vi "SeCrTs-Hardware Config.vi"() -> ()   [LabVIEW 2022 SP3]
uses:
  Controls/SeCrTs-Config.ctl
panel:
  in  "Signal list":bool
  out "Config":T1={"AO config"=[], "AI config"=[], "DI config"=[], "DO config"=[], "TC config"=[{"Channel_Name"="", "Channel_Number"="", "Pre_Scale_min"=0.0, "Pre_Scale_max"=0.0, "units"=4, " type"=7}], "ACC config"=[], "SG config"=[], "Strain Gauge Settings"={"poisson ratio"=0.3, "nominal gage resistance"=120.0, "gage factor"=2.08}, "Bridge Settings"={"voltage excitation value"=3.3, "voltage excitation source"=10200, "initial bridge voltage"=0.0, "lead wire resistance"=1.7, "strain configuration"=10271}, "Sample Rate"={"AI Sample Rate"=[], "AO Sample Rate"=[], "DI Sample Rate"=[], "TC Sample Rate"=[], "DO Sample Rate"=[], "SG Sample Rate"=[], "ACC Sample Rate"=[]}} {"Bridge Settings"."strain configuration" items=["Full Bridge I"=10183, "Full Bridge II"=10184, "Full Bridge III"=10185, "Half Bridge I"=10188, "Half Bridge II"=10189, "Quarter Bridge I"=10271, "Quarter Bridge II"=10272]; "Bridge Settings"."voltage excitation source" items=["Internal"=10200, "External"=10167, "None"=10230]; "ACC config"."Terminal configuration" items=["default"=-1, "RSE"=10083, "NRSE"=10078, "Differential"=10106, "Pseudodifferential"=12529]; "ACC config"."Sensitivity units" items=["mVolts/g"=12509, "Volts/g"=12510]; "TC config"."type" items=["J"=10072, "K"=10073, "N"=10077, "R"=10082, "S"=10085, "T"=10086, "B"=10047, "E"=10055]; "TC config"."units" items=["Deg C", "Deg F", "Kelvins", "Deg R", "From Custom Scale"]}
  in  "Cancel":bool
  in  "Load Configuration":bool
  in  "New configuration":bool
  in  "Save Config":bool
  in  "Tab Control":T2(tab)
  in  "DO Sample Rate":dbl[](array[numeric]) format="%#_g Hz"
  in  "DO config":T3(array[cluster])=[{"Channel_Name"="", "Channel_Number"="", "Default_Value"=FALSE, "Units"=FALSE}]
  out "DO Device List":string[](array[string])
  in  "DI Sample Rate":dbl[](array[numeric]) format="%#_g Hz"
  in  "DI config":T3(array[cluster])
  out "DI Device List":string[](array[string])
  in  "AO Sample Rate":dbl[](array[numeric]) format="%#_g Hz"
  in  "AO config":T4(array[cluster])
  out "AO Device List":string[](array[string])
  in  "AI Sample Rate":dbl[](array[numeric]) format="%#_g Hz"
  in  "AI config":T5(array[cluster])
  out "AI Device List":string[](array[string])
  in  "TC Sample Rate":dbl[](array[numeric]) format="%#_g Hz"
  in  "TC config":T6(array[cluster]) {"thermocouple type" items=["J"=10072, "K"=10073, "N"=10077, "R"=10082, "S"=10085, "T"=10086, "B"=10047, "E"=10055]; "units" items=["Deg C"=10143, "Deg F"=10144, "Kelvins"=10325, "Deg R"=10145, "From Custom Scale"=10065]}
  out "TC Device List":string[](array[string])
  in  "ACC Sample Rate":dbl[](array[numeric]) format="%#_g Hz"
  in  "ACC config":T7(array[cluster]) {"Sensitivity units" items=["mVolts/g"=12509, "Volts/g"=12510]; "Terminal configuration" items=["default"=-1, "RSE"=10083, "NRSE"=10078, "Differential"=10106, "Pseudodifferential"=12529]}
  out "ACC Device List":string[](array[string])
  out "SG Device List":string[](array[string])
  in  "SG Sample Rate":dbl[](array[numeric]) format="%#_g Hz"
  in  "SG config":T8(array[cluster])
  in  "SG Settings":T9={"gage factor"=2.08, "nominal gage \nresistance"=120.0, "poisson ratio"=0.3}
  in  "Bridge Settings":T10={"voltage excitation value"=3.3, "voltage excitation source"=10200, "initial bridge voltage"=0.0, "lead wire resistance"=1.7, "strain configuration"=10271} {"strain configuration" items=["Full Bridge I"=10183, "Full Bridge II"=10184, "Full Bridge III"=10185, "Half Bridge I"=10188, "Half Bridge II"=10189, "Quarter Bridge I"=10271, "Quarter Bridge II"=10272]; "voltage excitation source" items=["Internal"=10200, "External"=10167, "None"=10230]}
  # "DO_Channel_Name"
  # "DO_Channel_Number"
  # "Default Value"
  # "Invert?"
  # "DI_Channel_Name"
  # "DI_Channel_Number"
  # "Default Value"
  # "Invert?"
  # "AO_Channel_Name"
  # "AO_Channel_Number"
  # "Default Value"
  # "Units"
  # "AI_Channel_Name"
  # "AI_Channel_Number"
  # "Pre_Scale_min"
  # "Pre_Scale_max"
  # "Scale_min"
  # "Scale_max"
  # "Units"
  # "TC_Channel_Name"
  # "TC_Channel_Number"
  # "Max_Value"
  # "Units"
  # "Type"
  # "Min_Value"
  # "ACC_Channel_Name"
  # "ACC_Channel_Number"
  # "Min_Value"
  # "Max_Value"
  # "Terminal Config"
  # "Sensitivity"
  # "Sensitivity Units"
  # "SG_Channel_Name"
  # "SG_Channel_Number"
  # "Min_Value"
  # "Max_Value"
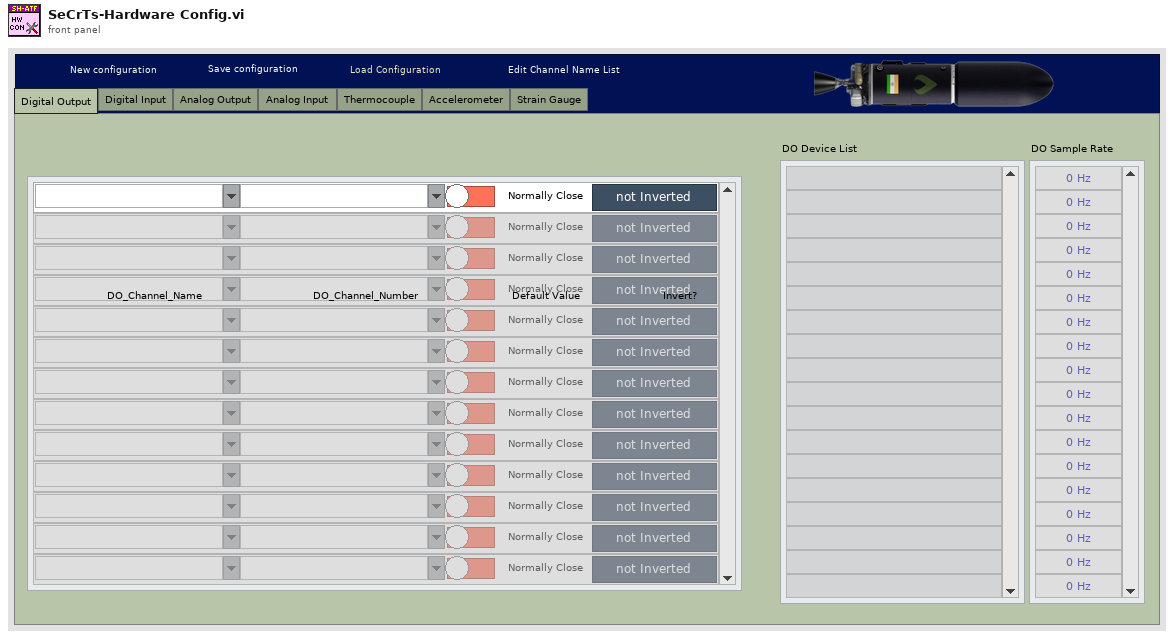
[diagram p1: front panel]
types:
  T1 = typedef "SeCrTs-Config.ctl" = cluster{"AO config":cluster{"Channel_Name":string, "Channel_Number":string, "Default_Value":dbl, "Units":string}[], "AI config":cluster{"Channel_Name":string, "Channel_Number":string, "Pre_Scale_min":dbl, "Pre_Scale_max":dbl, "Sensor_min":dbl, "Sensor_max":dbl, "Units":string}[], "DI config":cluster{"Channel_Name":string, "Channel_Number":string, "Default_Value":bool, "DI invert?":bool}[], "DO config":cluster{"Channel_Name":string, "Channel_Number":string, "Default_Value":bool, "DO invert?":bool}[], "TC config":cluster{"Channel_Name":string, "Channel_Number":string, "Pre_Scale_min":dbl, "Pre_Scale_max":dbl, "units":i32, " type":i32}[], "ACC config":cluster{"Channel_Name":string, "Channel_Number":string, "Pre_Scale_min":dbl, "Pre_Scale_max":dbl, "Terminal configuration":i32, "Sensitivity":dbl, "Sensitivity units":i32}[], "SG config":cluster{"Channel_Name":string, "Channel_Number":string, "Pre_Scale_min":dbl, "Pre_Scale_max":dbl}[], "Strain Gauge Settings":cluster{"poisson ratio":dbl, "nominal gage resistance":dbl, "gage factor":dbl}, "Bridge Settings":cluster{"voltage excitation value":dbl, "voltage excitation source":i32, "initial bridge voltage":dbl, "lead wire resistance":dbl, "strain configuration":i32}, "Sample Rate":cluster{"AI Sample Rate":dbl[], "AO Sample Rate":dbl[], "DI Sample Rate":dbl[], "TC Sample Rate":dbl[], "DO Sample Rate":dbl[], "SG Sample Rate":dbl[], "ACC Sample Rate":dbl[]}}
  T2 = enum32{"Digital Output", "Digital Input", "Analog Output", "Analog Input ", "Thermocouple", "Accelerometer", "Strain Gauge"}
  T3 = cluster{"Channel_Name":string, "Channel_Number":string, "Default_Value":bool, "Units":bool}[]
  T4 = cluster{"Channel_Name":string, "Channel_Number":string, "Default_Value":dbl, "Units":string}[]
  T5 = cluster{"Channel_Name":string, "Channel_Number":string, "Pre_Scale_min":dbl, "Pre_Scale_max":dbl, "Sensor_min":dbl, "Sensor_max":dbl, "Units":string}[]
  T6 = cluster{"Channel_Name":string, "Channel_Number":string, "Pre_Scale_min":dbl, "Pre_Scale_max":dbl, "units":i32, "thermocouple type":i32}[]
  T7 = cluster{"Channel_Name":string, "Channel_Number":string, "Pre_Scale_min":dbl, "Pre_Scale_max":dbl, "Terminal configuration":i32, "Sensitivity":dbl, "Sensitivity units":i32}[]
  T8 = cluster{"Channel_Name":string, "Channel_Number":string, "Pre_Scale_min":dbl, "Pre_Scale_max":dbl}[]
  T9 = cluster{"gage factor":dbl, "nominal gage \nresistance":dbl, "poisson ratio":dbl}
  T10 = cluster{"voltage excitation value":dbl, "voltage excitation source":i32, "initial bridge voltage":dbl, "lead wire resistance":dbl, "strain configuration":i32}
  T11 = cluster{"Device List":cluster{"AO Cards":tag[], "AI Cards":tag[], "DI Cards":tag[], "DO Cards":tag[]}, "Channel List":cluster{"AI Channel list":tag[], "AO Channel list":tag[], "DO Channel list ":tag[], "DI Channel list":tag[]}}
  T12 = cluster{"Channel List":cluster{"AI Channel list":tag[], "AO Channel list":tag[], "DO Channel list ":tag[], "DI Channel list":tag[]}, "Device List":cluster{"AO Cards":tag[], "AI Cards":tag[], "DI Cards":tag[], "DO Cards":tag[]}}
  T13 = cluster{"Data":T1, "path":path, "Name ref":refnum<vi>[], "Names":string[][], "Signal path":path, "SR":cluster{"AI Sample Rate":dbl[], "AO Sample Rate":dbl[], "DI Sample Rate":dbl[], "TC Sample Rate":dbl[], "DO Sample Rate":dbl[], "SG Sample Rate":dbl[], "ACC Sample Rate":dbl[]}, "Device List":cluster{"AO Cards":tag[], "AI Cards":tag[], "DI Cards":tag[], "DO Cards":tag[]}}
  T14 = typedef "SeCrTs-file folder ctl.ctl" = cluster{"Datalog path":path, "Configuration path":path, "Signal list path":path, "Sub vi's":path, "Authentication":path, "Sequence":path, "Event Log":path, "CS Error log":path, "RT Error Log":path}
  T15 = cluster{"AI":string[], "DI":string[], "DO":string[], "SG":string[], "AO":string[], "TC":string[], "ACC":string[]}
  T16 = cluster{"AI Channel list":tag[], "AO Channel list":tag[], "DO Channel list ":tag[], "DI Channel list":tag[]}
  T17 = cluster{"AO Cards":tag[], "AI Cards":tag[], "DI Cards":tag[], "DO Cards":tag[]}
  T18 = cluster{"AI Sample Rate":dbl[], "AO Sample Rate":dbl[], "DI Sample Rate":dbl[], "TC Sample Rate":dbl[], "DO Sample Rate":dbl[], "SG Sample Rate":dbl[], "ACC Sample Rate":dbl[]}
  T19 = enum16{"open", "replace", "create", "open or create", "replace or create", "replace or create with confirmation"}
  T20 = enum32{"Invalid", "Standard", "Closed", "Hidden", "Minimized", "Maximized"}
  T21 = cluster{"Channel_Name":string, "Channel_Number":string, "Default_Value":bool, "DI invert?":bool}[]
  T22 = cluster{"Channel_Name":string, "Channel_Number":string, "Default_Value":bool, "DO invert?":bool}[]
  T23 = cluster{"Channel_Name":string, "Channel_Number":string, "Pre_Scale_min":dbl, "Pre_Scale_max":dbl, "units":i32, " type":i32}[]
  T24 = cluster{"poisson ratio":dbl, "nominal gage resistance":dbl, "gage factor":dbl}
  T25 = cluster{"Channel_Name":string, "Channel_Number":string}
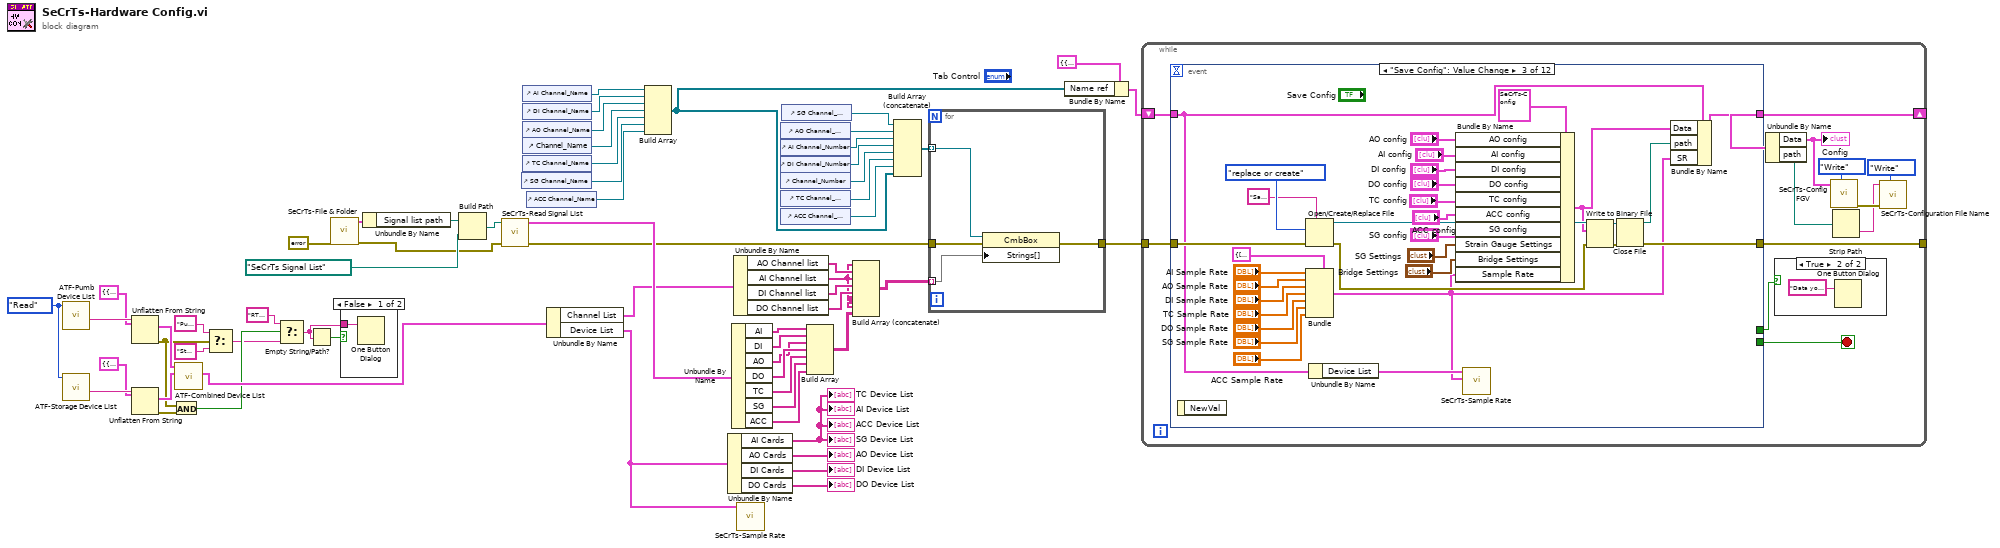
[diagram p0: block diagram]
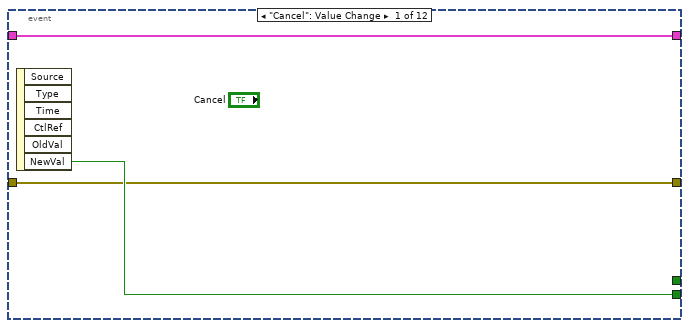
[diagram p4: hidden frame]
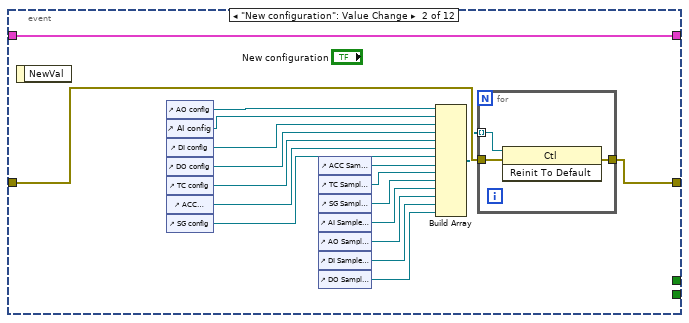
[diagram p5: hidden frame]
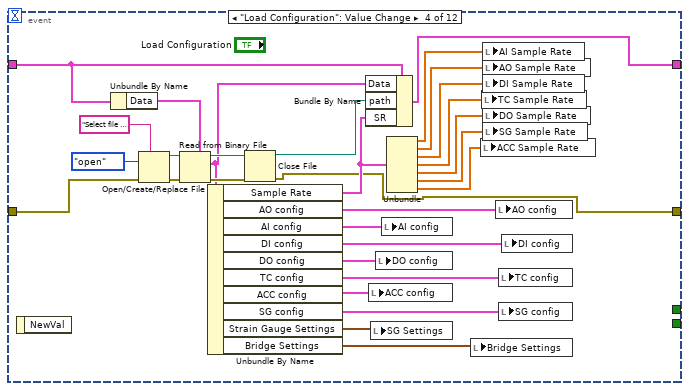
[diagram p6: hidden frame]
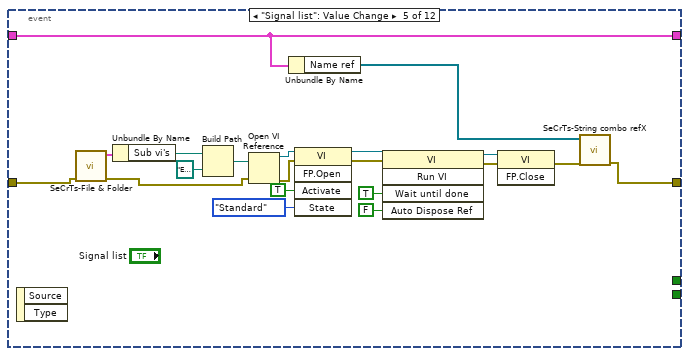
[diagram p7: hidden frame]
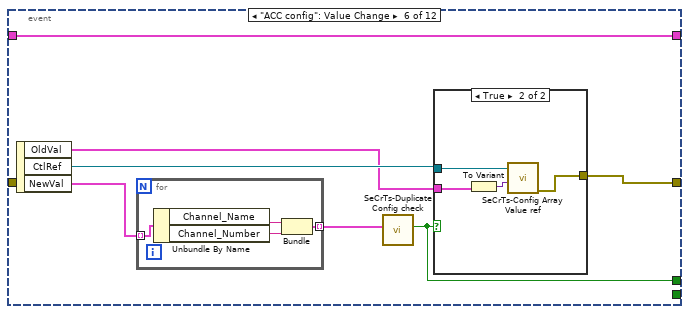
[diagram p8: hidden frame]
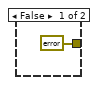
[diagram p9: hidden frame]
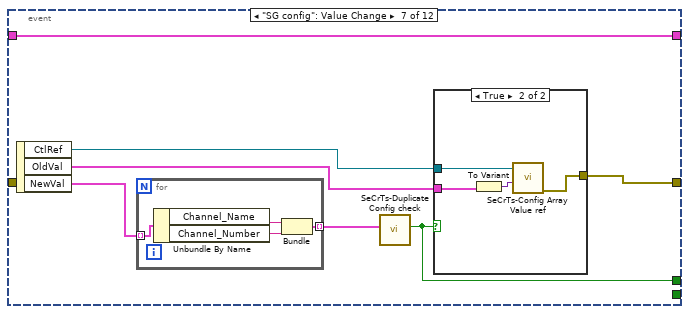
[diagram p10: hidden frame]
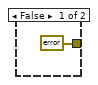
[diagram p11: hidden frame]
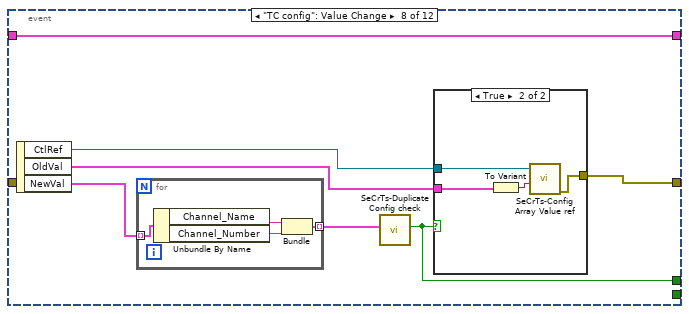
[diagram p12: hidden frame]
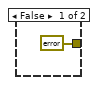
[diagram p13: hidden frame]
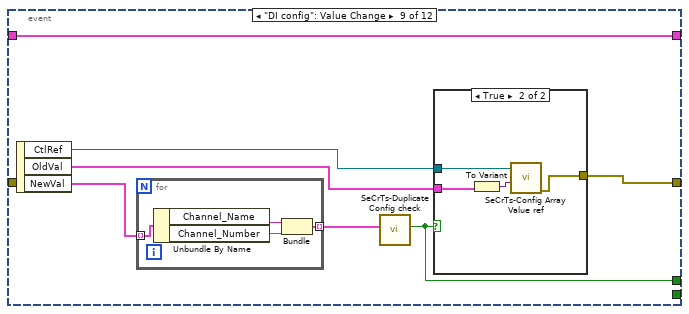
[diagram p14: hidden frame]
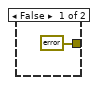
[diagram p15: hidden frame]
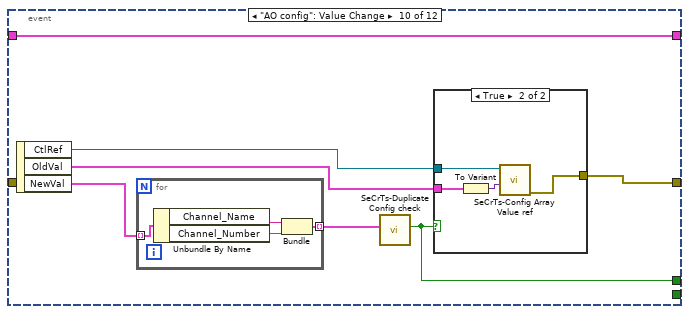
[diagram p16: hidden frame]
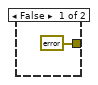
[diagram p17: hidden frame]
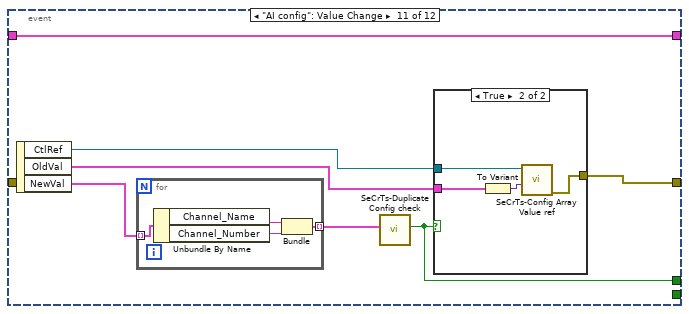
[diagram p18: hidden frame]
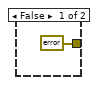
[diagram p19: hidden frame]
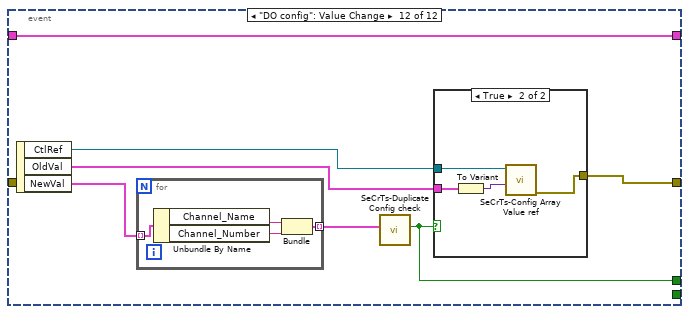
[diagram p20: hidden frame]
diagram:
  w16 = enum16{"Read", "Write", "Clear"}."Read" ("Enum")
  n1 = call "ATF-Pumb Device List.vi"("Enum"=w16) -> ("DL"=w15:string)  [unwired: 10 in]
  n2 = call "ATF-Storage Device List.vi"("Enum"=w16) -> ("DL"=w14:string)  [unwired: 10 in]
  n3 = Unflatten From String(type=T11 {"Device List"={"AO Cards"=[], "AI Cards"=[], "DI Cards"=[], "DO Cards"=[]}, "Channel List"={"AI Channel list"=[], "AO Channel list"=[], "DO Channel list "=[], "DI Channel list"=[]}}, binary string=w15) -> (value=w11:T11, error out=w6:errorcluster)  [unwired: 3 in, 1 out]
  n4 = Unflatten From String(type=T12 {"Channel List"={"AI Channel list"=[], "AO Channel list"=[], "DO Channel list "=[], "DI Channel list"=[]}, "Device List"={"AO Cards"=[], "AI Cards"=[], "DI Cards"=[], "DO Cards"=[]}}, binary string=w14) -> (value=w10:T12, error out=w9:errorcluster)  [unwired: 3 in, 1 out]
  n5 = And(x=w6, y=w9) -> (x .and. y?=w8:bool)
  n6 = call "ATF-Combined Device List.vi"("Storage"=w10, "Pump"=w11) -> ("Combined Device list"=w17:T12)  [unwired: 9 in]
  n7 = Select(t="Pump has heen not connected!" ("DL"), s=w6, f="Storage has heen not connected!" ("DL")) -> (s? t:f=w3:string)
  n8 = Select(t="RT has heen not connected!" ("DL"), s=w8, f=w3) -> (s? t:f=w2:string)
  n9 = Empty String/Path?(string/path=w2) -> (empty?=w1:bool)
  n10 = call "SeCrTs-File & Folder.vi"("error in (no error)"=errorcluster {"status"=FALSE, "code"=0, "source"=""} ("error in")) -> ("error out"=w42:errorcluster, "File Output"=w48:T14)  [unwired: 9 in]
  n11 = case shown="False" w1 {
    tunnel: w2 -> [w64 _]
    frame False {
      n12 = One Button Dialog(message=w64) -> ()  [unwired: 1 in, 1 out]
    }
    frame True {
    }
  }
  n13 = Unbundle By Name(w48) -> ("Signal list path"=w47:path)
  n14 = Build Path(base path=w47, name or relative path=path "SeCrTs Signal List") -> (appended path=w21:path)
  n15 = call "SeCrTs-Read Signal List.vi"("error in"=w42, "file path (use dialog)"=w21) -> ("error out"=w20:errorcluster, "Names"=w41:T15)  [unwired: 8 in]
  n16 = control-ref of="SG Channel_Name"() -> (w27:refnum<vi>)
  n17 = control-ref of="AI Channel_Name"() -> (w45:refnum<vi>)
  n18 = control-ref of="DI Channel_Name"() -> (w44:refnum<vi>)
  n19 = control-ref of="AO Channel_Name"() -> (w29:refnum<vi>)
  n20 = control-ref of="Channel_Name"() -> (w28:refnum<vi>)
  n21 = control-ref of="TC Channel_Name"() -> (w43:refnum<vi>)
  n22 = control-ref of="ACC Channel_Name"() -> (w26:refnum<vi>)
  n23 = Unbundle By Name(w17) -> ("Channel List"=w18:T16, "Device List"=w19:T17)
  n24 = Build Array(w45, w44, w29, w28, w43, w27, w26) -> (w30:refnum<vi>[])
  n25 = Unbundle By Name(w19) -> ("AI Cards"=→"AI Device List" →"TC Device List" →"ACC Device List" →"SG Device List":tag[], "AO Cards"=→"AO Device List":tag[], "DI Cards"=→"DI Device List":tag[], "DO Cards"=→"DO Device List":tag[])
  n26 = Unbundle By Name(w41) -> ("AI"=w40:string[], "DI"=w39:string[], "AO"=w34:string[], "DO"=w38:string[], "TC"=w37:string[], "SG"=w36:string[], "ACC"=w35:string[])
  n27 = Unbundle By Name(w18) -> ("AO Channel list"=w51:tag[], "AI Channel list"=w50:tag[], "DI Channel list"=w58:tag[], "DO Channel list"=w57:tag[])
  n28 = call "SeCrTs-Sample Rate.vi"("Device List"=w19) -> ()  [unwired: 11 in]
  n29 = control-ref of="AO Channel_Number"() -> (w63:refnum<vi>)
  n30 = control-ref of="AI Channel_Number"() -> (w62:refnum<vi>)
  n31 = control-ref of="DI Channel_Number"() -> (w61:refnum<vi>)
  n32 = control-ref of="Channel_Number"() -> (w60:refnum<vi>)
  n33 = control-ref of="TC Channel_Number"() -> (w54:refnum<vi>)
  n34 = control-ref of="ACC Channel_Number"() -> (w53:refnum<vi>)
  n35 = control-ref of="SG Channel_Number"() -> (w52:refnum<vi>)
  n36 = Build Array(w40, w39, w34, w38, w37, w36, w35) -> (w33:string[][])
  n37 = Build Array (concatenate)(w50, w51, w50, w58, w57, w50, w50, w33) -> (w56:string[][])
  n38 = Build Array (concatenate)(w52, w63, w62, w61, w60, w54, w53, w30) -> (w59:refnum<vi>[])
  n39 = for {
    tunnel: w59 -> [w68] mode=indexing
    tunnel: w56 -> [w65] mode=indexing
    tunnel: [w67] -> w55
    tunnel: w20 -> [w66]
    n40 = property class="CmbBox"(reference=w68, error in=w66, "Strings[]"=w65) -> (error out=w67:errorcluster)  [unwired: 1 out]
  }
  n41 = Bundle By Name(cluster=T13 {"Data"={"AO config"=[], "AI config"=[], "DI config"=[], "DO config"=[], "TC config"=[{"Channel_Name"="", "Channel_Number"="", "Pre_Scale_min"=0.0, "Pre_Scale_max"=0.0, "units"=4, " type"=7}], "ACC config"=[], "SG config"=[], "Strain Gauge Settings"={"poisson ratio"=0.3, "nominal gage resistance"=120.0, "gage factor"=2.08}, "Bridge Settings"={"voltage excitation value"=3.3, "voltage excitation source"=10200, "initial bridge voltage"=0.0, "lead wire resistance"=1.7, "strain configuration"=10271}, "Sample Rate"={"AI Sample Rate"=[], "AO Sample Rate"=[], "DI Sample Rate"=[], "TC Sample Rate"=[], "DO Sample Rate"=[], "SG Sample Rate"=[], "ACC Sample Rate"=[]}}, "path"=path "", "Name ref"=[], "Names"=[], "Signal path"=path "", "SR"={"AI Sample Rate"=[], "AO Sample Rate"=[], "DI Sample Rate"=[], "TC Sample Rate"=[], "DO Sample Rate"=[], "SG Sample Rate"=[], "ACC Sample Rate"=[]}, "Device List"={"AO Cards"=["PXI1Slot2"], "AI Cards"=["cDAQ1Mod1", "cDAQ1Mod2", "cDAQ1Mod3", "cDAQ1Mod4"], "DI Cards"=["cDAQ1Mod5", "PXI1Slot2", "PXI1Slot3"], "DO Cards"=["cDAQ1Mod5", "PXI1Slot2", "PXI1Slot3"]}}, "Name ref"=w30) -> (w32:T13)
  n42 = while {
    shift-right: [w76] -> _
    shift-left: w32 -> [w77]
    tunnel: w55 -> [w79]
    tunnel: [w78] -> _
    stop <- w80 stop-if-true
    n43 = event shown="[2] \"Save Config\": Value Change" {
      selector: _ -> [_ _ _ _ _ _ _ _ _ _ _ _]
      dyn-events: _ -> [_ _ _ _ _ _ _ _ _ _ _ _]
      timeout: _ -> [_ _ _ _ _ _ _ _ _ _ _ _]
      tunnel: [w83 _ _ _ _ _ _ _ _ _ _ _] -> w80
      tunnel: w79 -> [w82 w102 w137 w167 w187 _ _ _ _ _ _ _]
      tunnel: [w82 w101 w133 w144 w169 w189 w207 w223 w239 w255 w271 w287] -> w78
      tunnel: w77 -> [w84 w100 w109 w158 w172 w194 w210 w226 w242 w258 w274 w290]
      tunnel: [w84 w100 w125 w159 w172 w194 w210 w226 w242 w258 w274 w290] -> w76
      tunnel: [_ _ _ _ _ w188 w204 w220 w236 w252 w268 w284] -> w72
      event "Cancel": Value Change {
        n44 = event-data() -> ("NewVal"=w83:bool)  [unwired: 1 in, 5 out]
      }
      event "New configuration": Value Change {
        n45 = event-data() -> ()  [unwired: 1 in, 1 out]
        n46 = control-ref of="AO config"() -> (w95:refnum<vi>)
        n47 = control-ref of="AI config"() -> (w96:refnum<vi>)
        n48 = control-ref of="DI config"() -> (w97:refnum<vi>)
        n49 = control-ref of="DO config"() -> (w98:refnum<vi>)
        n50 = control-ref of="TC config"() -> (w94:refnum<vi>)
        n51 = control-ref of="ACC config"() -> (w93:refnum<vi>)
        n52 = control-ref of="SG config"() -> (w92:refnum<vi>)
        n53 = control-ref of="ACC Sample Rate"() -> (w91:refnum<vi>)
        n54 = control-ref of="TC Sample Rate"() -> (w90:refnum<vi>)
        n55 = control-ref of="SG Sample Rate"() -> (w89:refnum<vi>)
        n56 = control-ref of="AI Sample Rate"() -> (w88:refnum<vi>)
        n57 = control-ref of="AO Sample Rate"() -> (w87:refnum<vi>)
        n58 = control-ref of="DI Sample Rate"() -> (w86:refnum<vi>)
        n59 = control-ref of="DO Sample Rate"() -> (w85:refnum<vi>)
        n60 = Build Array(w95, w96, w97, w98, w94, w93, w92, w91, w90, w89, w88, w87, w86, w85) -> (w99:refnum<vi>[])
        n61 = for {
          tunnel: w99 -> [w105] mode=indexing
          tunnel: w102 -> [w104]
          tunnel: [w103] -> w101
          n62 = invoke class="Ctl" method="Reinit To Default"(reference=w105, error in=w104) -> (error out=w103:errorcluster)  [unwired: 1 in, 2 out]
        }
      }
      event "Save Config": Value Change {
        n63 = event-data() -> ()  [unwired: 1 in, 1 out]
        n64 = Open/Create/Replace File(error in=w137, prompt="Save Changes", operation (0:open)=T19."replace or create") -> (refnum out=w132:refnum<file>, error out=w136:errorcluster)  [unwired: 3 in, 1 out]
        n65 = Bundle(cluster=T18 {"AI Sample Rate"=[], "AO Sample Rate"=[], "DI Sample Rate"=[], "TC Sample Rate"=[], "DO Sample Rate"=[], "SG Sample Rate"=[], "ACC Sample Rate"=[]} ("Sample Rate"), "AI Sample Rate"="AI Sample Rate", "AO Sample Rate"="AO Sample Rate", "DI Sample Rate"="DI Sample Rate", "TC Sample Rate"="TC Sample Rate", "DO Sample Rate"="DO Sample Rate", "SG Sample Rate"="SG Sample Rate", "ACC Sample Rate"="ACC Sample Rate") -> (w107:T18)
        n66 = Unbundle By Name(w109) -> ("Device List"=w108:T17)
        n67 = Bundle By Name(cluster=T1 {"AO config"=[], "AI config"=[], "DI config"=[], "DO config"=[], "TC config"=[{"Channel_Name"="", "Channel_Number"="", "Pre_Scale_min"=0.0, "Pre_Scale_max"=0.0, "units"=4, " type"=7}], "ACC config"=[], "SG config"=[], "Strain Gauge Settings"={"poisson ratio"=0.3, "nominal gage resistance"=120.0, "gage factor"=2.08}, "Bridge Settings"={"voltage excitation value"=3.3, "voltage excitation source"=10200, "initial bridge voltage"=0.0, "lead wire resistance"=1.7, "strain configuration"=10271}, "Sample Rate"={"AI Sample Rate"=[], "AO Sample Rate"=[], "DI Sample Rate"=[], "TC Sample Rate"=[], "DO Sample Rate"=[], "SG Sample Rate"=[], "ACC Sample Rate"=[]}} ("Data"), "AO config"="AO config", "AI config"="AI config", "DI config"="DI config", "DO config"="DO config", "TC config"="TC config", "ACC config"="ACC config", "SG config"="SG config", "Strain Gauge Settings"="SG Settings", "Bridge Settings"="Bridge Settings", "Sample Rate"=w107) -> (w106:T1)
        n68 = call "SeCrTs-Sample Rate.vi"("Sample Rate"=w107, "Device List"=w108) -> ()  [unwired: 10 in]
        n69 = Write to Binary File(file (use dialog)=w132, data=w106, error in=w136) -> (refnum out=w135:refnum<file>, error out=w134:errorcluster)  [unwired: 3 in, 1 out]
        n70 = Close File(refnum=w135, error in=w134) -> (path=w120:path, error out=w133:errorcluster)
        n71 = Bundle By Name(cluster=w109, "Data"=w106, "path"=w120, "SR"=w107) -> (w125:T13)
      }
      event "Load Configuration": Value Change {
        n72 = event-data() -> ()  [unwired: 1 in, 1 out]
        n73 = Unbundle By Name(w158) -> ("Data"=w160:T1)
        n74 = Open/Create/Replace File(error in=w167, prompt="Select file to load", operation (0:open)=T19."open") -> (refnum out=w163:refnum<file>, error out=w166:errorcluster)  [unwired: 3 in, 1 out]
        n75 = Read from Binary File(5:w160, 8:w166, 11:w163) -> (0:w164:errorcluster, 2:w157:T1, 3:w165:refnum<file>)  [unwired: 3 in, 1 out]
        n76 = Unbundle By Name(w157) -> ("Sample Rate"=w146:T18, "AO config"=w156:T4, "AI config"=w155:T5, "DI config"=w154:T21, "DO config"=w153:T22, "TC config"=w152:T23, "ACC config"=w151:T7, "SG config"=w150:T8, "Strain Gauge Settings"=w148:T24, "Bridge Settings"=w147:T10)
        n77 = Close File(refnum=w165, error in=w164) -> (path=w149:path, error out=w144:errorcluster)
        n78 = Bundle By Name(cluster=w158, "Data"=w157, "path"=w149, "SR"=w146) -> (w159:T13)
        n79 = local write "ACC config"(w151) -> ()
        n80 = local write "SG Settings"(w148) -> ()
        n81 = local write "DO config"(w153) -> ()
        n82 = local write "AI config"(w155) -> ()
        n83 = Unbundle(w146) -> ("AI Sample Rate"=w145:dbl[], "AO Sample Rate"=w143:dbl[], "DI Sample Rate"=w142:dbl[], "TC Sample Rate"=w141:dbl[], "DO Sample Rate"=w140:dbl[], "SG Sample Rate"=w139:dbl[], "ACC Sample Rate"=w138:dbl[])
        n84 = local write "Bridge Settings"(w147) -> ()
        n85 = local write "ACC Sample Rate"(w138) -> ()
        n86 = local write "TC Sample Rate"(w141) -> ()
        n87 = local write "AI Sample Rate"(w145) -> ()
        n88 = local write "AO Sample Rate"(w143) -> ()
        n89 = local write "DI Sample Rate"(w142) -> ()
        n90 = local write "DO Sample Rate"(w140) -> ()
        n91 = local write "SG Sample Rate"(w139) -> ()
        n92 = local write "AO config"(w156) -> ()
        n93 = local write "TC config"(w152) -> ()
        n94 = local write "SG config"(w150) -> ()
        n95 = local write "DI config"(w154) -> ()
      }
      event "Signal list": Value Change {
        n96 = event-data() -> ()  [unwired: 1 in, 2 out]
        n97 = call "SeCrTs-File & Folder.vi"("error in (no error)"=w187) -> ("error out"=w183:errorcluster, "File Output"=w186:T14)  [unwired: 9 in]
        n98 = Unbundle By Name(w186) -> ("Sub vi's"=w185:path)
        n99 = Build Path(base path=w185, name or relative path=path "Edit Channel Name list.vi") -> (appended path=w168:path)
        n100 = Open VI Reference(vi path=w168, error in (no error)=w183) -> (vi reference=w174:refnum<vi>, error out=w173:errorcluster)  [unwired: 4 in]
        n101 = Unbundle By Name(w172) -> ("Name ref"=w171:refnum<vi>[])
        n102 = invoke class="VI" method="FP.Open"(reference=w174, error in=w173, "Activate"=TRUE ("Activate?"), "State"=T20."Standard") -> (reference out=w182:refnum<vi>, error out=w181:errorcluster)  [unwired: 1 in, 3 out]
        n103 = invoke class="VI" method="Run VI"(reference=w182, error in=w181, "Wait until done"=TRUE ("Wait Until Done"), "Auto Dispose Ref"=FALSE ("Auto Dispose Reference")) -> (reference out=w180:refnum<vi>, error out=w179:errorcluster)  [unwired: 1 in, 3 out]
        n104 = invoke class="VI" method="FP.Close"(reference=w180, error in=w179) -> (error out=w170:errorcluster)  [unwired: 1 in, 2 out]
        n105 = call "SeCrTs-String combo refX.vi"("error out"=w170, "Ctrl ref"=w171) -> ("error out 2"=w169:errorcluster)  [unwired: 9 in]
      }
      event "ACC config": Value Change {
        n106 = event-data() -> ("OldVal"=w190:T7, "CtlRef"=w191:refnum<vi>, "NewVal"=w193:T7)  [unwired: 1 in]
        n107 = for {
          tunnel: w193 -> [w198] mode=indexing
          tunnel: [w195] -> w192 mode=indexing
          n108 = Unbundle By Name(w198) -> ("Channel_Name"=w196:string, "Channel_Number"=w197:string)
          n109 = Bundle("Channel_Name"=w196, "Channel_Number"=w197) -> (w195:T25)  [unwired: 1 in]
        }
        n110 = call "SeCrTs-Duplicate Config check.vi"("Data in"=w192) -> ("Channel list indication"=w188:bool)  [unwired: 10 in]
        n111 = case shown="True" w188 {
          tunnel: w191 -> [_ w202]
          tunnel: w190 -> [_ w201]
          tunnel: [errorcluster {"status"=FALSE, "code"=0, "source"=""} ("error out") w200] -> w189
          frame False {
          }
          frame True {
            n112 = To Variant(anything=w201) -> (Variant=w203:variant)
            n113 = call "SeCrTs-Config Array Value ref.vi"("Value"=w203, "Array in"=w202) -> ("error out"=w200:errorcluster)  [unwired: 9 in]
          }
        }
      }
      event "SG config": Value Change {
        n114 = event-data() -> ("CtlRef"=w206:refnum<vi>, "OldVal"=w205:T8, "NewVal"=w209:T8)  [unwired: 1 in]
        n115 = for {
          tunnel: w209 -> [w214] mode=indexing
          tunnel: [w211] -> w208 mode=indexing
          n116 = Unbundle By Name(w214) -> ("Channel_Name"=w212:string, "Channel_Number"=w213:string)
          n117 = Bundle("Channel_Name"=w212, "Channel_Number"=w213) -> (w211:T25)  [unwired: 1 in]
        }
        n118 = call "SeCrTs-Duplicate Config check.vi"("Data in"=w208) -> ("Channel list indication"=w204:bool)  [unwired: 10 in]
        n119 = case shown="True" w204 {
          tunnel: w206 -> [_ w218]
          tunnel: w205 -> [_ w217]
          tunnel: [errorcluster {"status"=FALSE, "code"=0, "source"=""} ("error out") w216] -> w207
          frame False {
          }
          frame True {
            n120 = To Variant(anything=w217) -> (Variant=w219:variant)
            n121 = call "SeCrTs-Config Array Value ref.vi"("Value"=w219, "Array in"=w218) -> ("error out"=w216:errorcluster)  [unwired: 9 in]
          }
        }
      }
      event "TC config": Value Change {
        n122 = event-data() -> ("CtlRef"=w222:refnum<vi>, "OldVal"=w221:T6, "NewVal"=w225:T6)  [unwired: 1 in]
        n123 = for {
          tunnel: w225 -> [w230] mode=indexing
          tunnel: [w227] -> w224 mode=indexing
          n124 = Unbundle By Name(w230) -> ("Channel_Name"=w228:string, "Channel_Number"=w229:string)
          n125 = Bundle("Channel_Name"=w228, "Channel_Number"=w229) -> (w227:T25)  [unwired: 1 in]
        }
        n126 = call "SeCrTs-Duplicate Config check.vi"("Data in"=w224) -> ("Channel list indication"=w220:bool)  [unwired: 10 in]
        n127 = case shown="True" w220 {
          tunnel: w222 -> [_ w234]
          tunnel: w221 -> [_ w233]
          tunnel: [errorcluster {"status"=FALSE, "code"=0, "source"=""} ("error out") w232] -> w223
          frame False {
          }
          frame True {
            n128 = To Variant(anything=w233) -> (Variant=w235:variant)
            n129 = call "SeCrTs-Config Array Value ref.vi"("Value"=w235, "Array in"=w234) -> ("error out"=w232:errorcluster)  [unwired: 9 in]
          }
        }
      }
      event "DI config": Value Change {
        n130 = event-data() -> ("CtlRef"=w238:refnum<vi>, "OldVal"=w237:T3, "NewVal"=w241:T3)  [unwired: 1 in]
        n131 = for {
          tunnel: w241 -> [w246] mode=indexing
          tunnel: [w243] -> w240 mode=indexing
          n132 = Unbundle By Name(w246) -> ("Channel_Name"=w244:string, "Channel_Number"=w245:string)
          n133 = Bundle("Channel_Name"=w244, "Channel_Number"=w245) -> (w243:T25)  [unwired: 1 in]
        }
        n134 = call "SeCrTs-Duplicate Config check.vi"("Data in"=w240) -> ("Channel list indication"=w236:bool)  [unwired: 10 in]
        n135 = case shown="True" w236 {
          tunnel: w238 -> [_ w250]
          tunnel: w237 -> [_ w249]
          tunnel: [errorcluster {"status"=FALSE, "code"=0, "source"=""} ("error out") w248] -> w239
          frame False {
          }
          frame True {
            n136 = To Variant(anything=w249) -> (Variant=w251:variant)
            n137 = call "SeCrTs-Config Array Value ref.vi"("Value"=w251, "Array in"=w250) -> ("error out"=w248:errorcluster)  [unwired: 9 in]
          }
        }
      }
      event "AO config": Value Change {
        n138 = event-data() -> ("CtlRef"=w254:refnum<vi>, "OldVal"=w253:T4, "NewVal"=w257:T4)  [unwired: 1 in]
        n139 = for {
          tunnel: w257 -> [w262] mode=indexing
          tunnel: [w259] -> w256 mode=indexing
          n140 = Unbundle By Name(w262) -> ("Channel_Name"=w260:string, "Channel_Number"=w261:string)
          n141 = Bundle("Channel_Name"=w260, "Channel_Number"=w261) -> (w259:T25)  [unwired: 1 in]
        }
        n142 = call "SeCrTs-Duplicate Config check.vi"("Data in"=w256) -> ("Channel list indication"=w252:bool)  [unwired: 10 in]
        n143 = case shown="True" w252 {
          tunnel: w254 -> [_ w267]
          tunnel: w253 -> [_ w265]
          tunnel: [errorcluster {"status"=FALSE, "code"=0, "source"=""} ("error out") w266] -> w255
          frame False {
          }
          frame True {
            n144 = To Variant(anything=w265) -> (Variant=w264:variant)
            n145 = call "SeCrTs-Config Array Value ref.vi"("Value"=w264, "Array in"=w267) -> ("error out"=w266:errorcluster)  [unwired: 9 in]
          }
        }
      }
      event "AI config": Value Change {
        n146 = event-data() -> ("CtlRef"=w270:refnum<vi>, "OldVal"=w269:T5, "NewVal"=w273:T5)  [unwired: 1 in]
        n147 = for {
          tunnel: w273 -> [w278] mode=indexing
          tunnel: [w275] -> w272 mode=indexing
          n148 = Unbundle By Name(w278) -> ("Channel_Name"=w276:string, "Channel_Number"=w277:string)
          n149 = Bundle("Channel_Name"=w276, "Channel_Number"=w277) -> (w275:T25)  [unwired: 1 in]
        }
        n150 = call "SeCrTs-Duplicate Config check.vi"("Data in"=w272) -> ("Channel list indication"=w268:bool)  [unwired: 10 in]
        n151 = case shown="True" w268 {
          tunnel: w270 -> [_ w282]
          tunnel: w269 -> [_ w281]
          tunnel: [errorcluster {"status"=FALSE, "code"=0, "source"=""} ("error out") w280] -> w271
          frame False {
          }
          frame True {
            n152 = To Variant(anything=w281) -> (Variant=w283:variant)
            n153 = call "SeCrTs-Config Array Value ref.vi"("Value"=w283, "Array in"=w282) -> ("error out"=w280:errorcluster)  [unwired: 9 in]
          }
        }
      }
      event "DO config": Value Change {
        n154 = event-data() -> ("CtlRef"=w286:refnum<vi>, "OldVal"=w285:T3, "NewVal"=w289:T3)  [unwired: 1 in]
        n155 = for {
          tunnel: w289 -> [w294] mode=indexing
          tunnel: [w291] -> w288 mode=indexing
          n156 = Unbundle By Name(w294) -> ("Channel_Name"=w292:string, "Channel_Number"=w293:string)
          n157 = Bundle("Channel_Name"=w292, "Channel_Number"=w293) -> (w291:T25)  [unwired: 1 in]
        }
        n158 = call "SeCrTs-Duplicate Config check.vi"("Data in"=w288) -> ("Channel list indication"=w284:bool)  [unwired: 10 in]
        n159 = case shown="True" w284 {
          tunnel: w286 -> [_ w299]
          tunnel: w285 -> [_ w297]
          tunnel: [errorcluster {"status"=FALSE, "code"=0, "source"=""} ("error out") w298] -> w287
          frame False {
          }
          frame True {
            n160 = To Variant(anything=w297) -> (Variant=w296:variant)
            n161 = call "SeCrTs-Config Array Value ref.vi"("Value"=w296, "Array in"=w299) -> ("error out"=w298:errorcluster)  [unwired: 9 in]
          }
        }
      }
    }
    n162 = Unbundle By Name(w76) -> ("Data"=w75:T1, "path"=w73:path)
    "Config" <- w75
    n163 = case shown="True" w72 {
      frame False {
      }
      frame True {
        n164 = One Button Dialog ("Warning")(message="Data you Entered is already Exist!") -> ()  [unwired: 1 in, 1 out]
      }
    }
    n165 = call "SeCrTs-Config FGV.vi"("Enum"=enum16{"Read", "Write"}."Write", "Data 2"=w75) -> ("error out"=w71:errorcluster)  [unwired: 8 in, 1 out]
    n166 = Strip Path(path=w73) -> (name=w70:string)  [unwired: 1 out]
    n167 = call "SeCrTs-Configuration File Name.vi"("Enum"=enum16{"Read", "Write"}."Write", "error in"=w71, "Phase code W"=w70) -> ()  [unwired: 7 in, 2 out]
  }
